vi "DELETE File Name.vi"   [LabVIEW 2013]
uses:
  Action.ctl
  Persistent Data FGV Selector.ctl
types:
  T1 = typedef "Persistent Data FGV Selector.ctl" = enum16{"Save Directory", "File Name"}
  T2 = typedef "Action.ctl" = enum16{"GET", "PUT", "DELETE"}
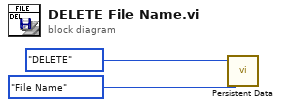
[diagram p0: block diagram]
diagram:
  n1 = call "Persistent Data.vi"("Persistent Data FGV Selector"=Persistent_Data_FGV_Selector."File Name", "Action"=Action."DELETE") -> ()  [unwired: 1 in, 1 out]
